vi "PMT imaging_ v2.vi"() -> ()   [LabVIEW 2012]
uses:
  <vilib>/DAQmx/write.llb/DAQmx Write (Analog 1D Wfm NChan NSamp).vi
  <vilib>/DAQmx/read.llb/DAQmx Read (Counter 1D U32 1Chan NSamp).vi
  <vilib>/DAQmx/create/channels.llb/DAQmx Create Channel (AO-Voltage-Basic).vi
  <vilib>/DAQmx/configure/timing.llb/DAQmx Timing (Sample Clock).vi
  <vilib>/DAQmx/configure/trigger.llb/DAQmx Start Trigger (Digital Edge).vi
  <vilib>/DAQmx/create/channels.llb/DAQmx Create Channel (CI-Count Edges).vi
  <vilib>/DAQmx/miscellaneous.llb/DAQmx Fill In Error Info.vi
  <resource>/objmgr/daqmx.rc
panel:
  in  "shift":i8
  in  "String":string
  out "Image original":T1(plugin-control)
  in  "Slices":i32
  in  "Step size(um)":dbl
  in  "Normalization":dbl=255.0
  out "Output":dbl[](array[numeric])
  out "size(s)":i32
  out "data":u32[](array[numeric])
  out "image normalize":T1(plugin-control)
  in  "Exp Time (s)":dbl=4.0
  in  "Y line":i32=512
  in  "Y step (um)":dbl=0.1
  in  "X step (um)":dbl=0.1
  in  "X pixel":i32=512
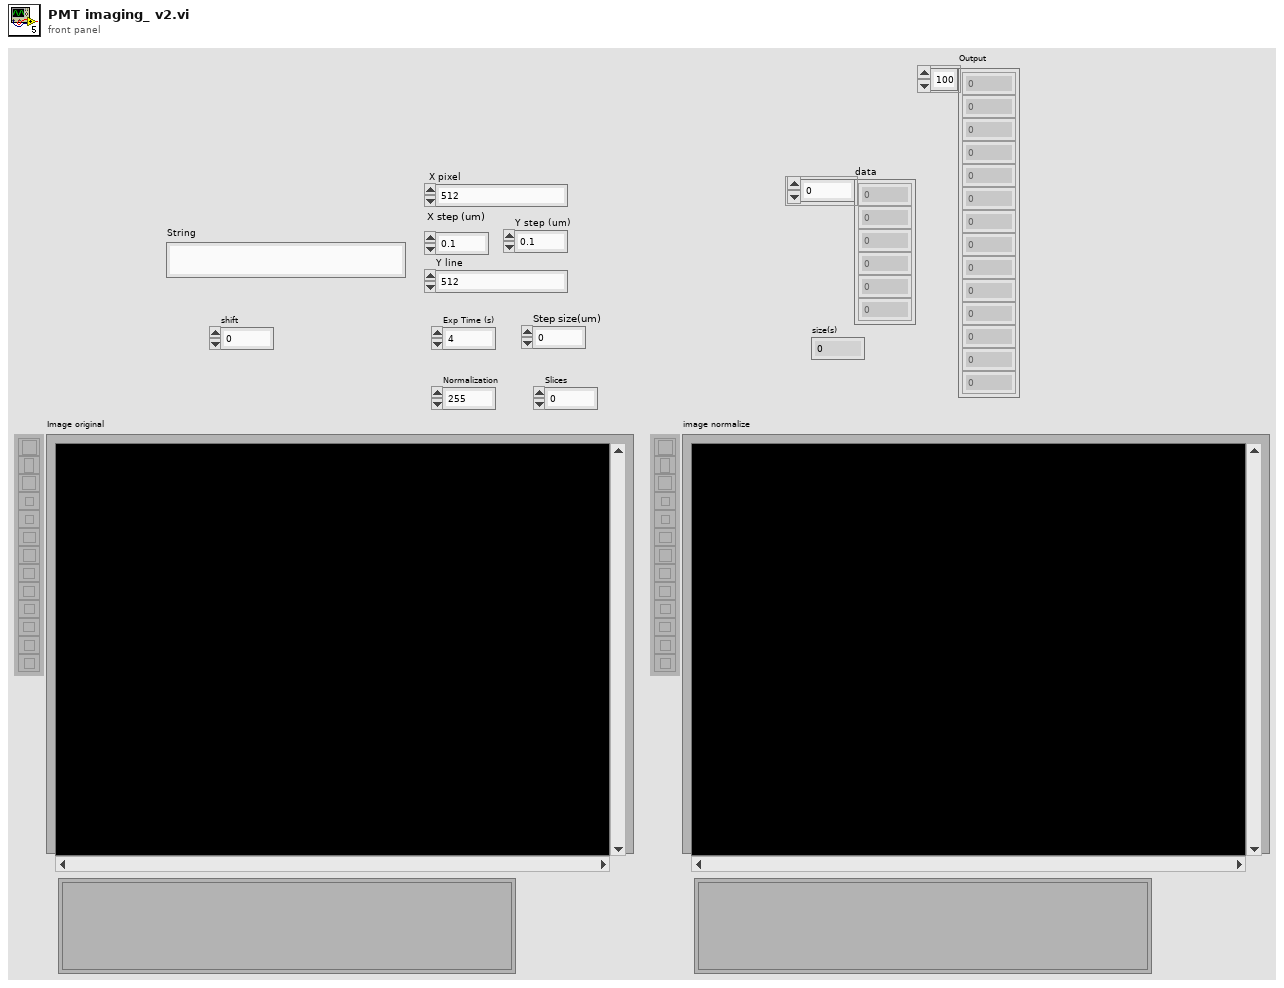
[diagram p1: front panel]
types:
  T1 = typedef "IMAQ Image.ctl" = refnum<image>
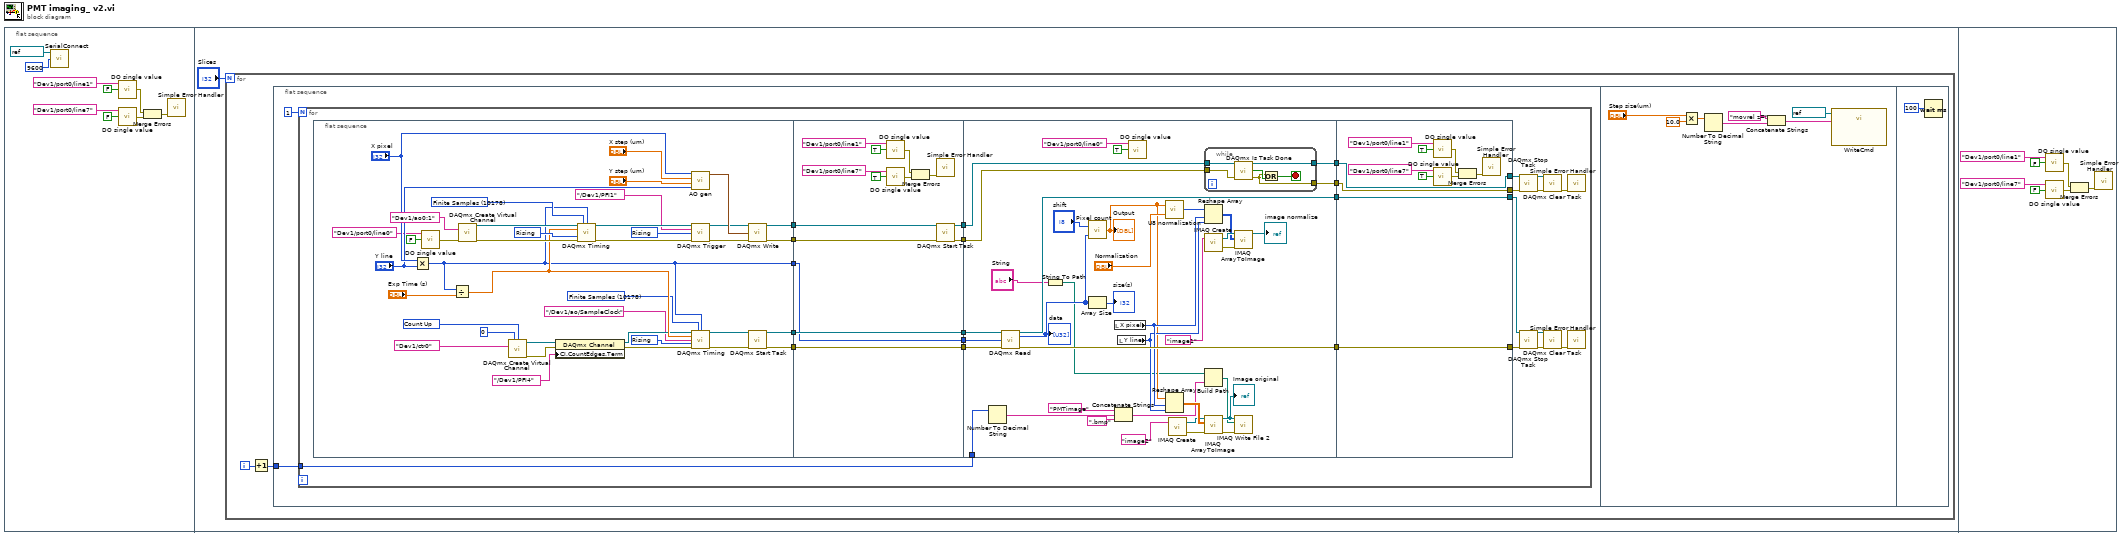
[diagram p0: block diagram]
diagram:
  n1 = flat-sequence {
    frame #0 {
      n2 = call "SerialConnect.vi"("baud rate (9600)"=u32 9600, "VISA resource name"=refnum<visa-resource-name> "COM1") -> ()  [unwired: 1 in, 3 out]
      n3 = call "DO single value.vi"("data"=FALSE, "lines"=tag "Dev1/port0/line1") -> ("error out"=w2:errorcluster)  [unwired: 1 in]
      n4 = call "DO single value.vi"("data"=FALSE, "lines"=tag "Dev1/port0/line7") -> ("error out"=w1:errorcluster)  [unwired: 1 in]
      n5 = Merge Errors(w2, w1) -> (w3:errorcluster)
      n6 = call <vilib>:"Simple Error Handler.vi"("error in (no error)"=w3) -> ()  [unwired: 4 in, 5 out]
    }
    frame #1 {
      n7 = for {
        N: "Slices" -> [_]
        i -> [w12]
        n8 = Increment(x=w12) -> (x+1=w11:i32)
        n9 = flat-sequence {
          tunnel: w11 -> [w13]
          frame #0 {
            n10 = for {
              N: 1 -> [_]
              tunnel: w13 -> [w15]
              n11 = flat-sequence {
                tunnel: [w61] -> w31
                tunnel: [w60] -> w30
                tunnel: [w51] -> w29
                tunnel: [w50] -> w28
                tunnel: [w49] -> w27
                tunnel: [w92] -> w24
                tunnel: [w91] -> w23
                tunnel: [w90] -> w22
                tunnel: [w89] -> w21
                tunnel: [w88] -> w20
                tunnel: w27 -> [w88]
                tunnel: w28 -> [w86]
                tunnel: w29 -> [w87]
                tunnel: w30 -> [w91]
                tunnel: w31 -> [w92]
                tunnel: w24 -> [w124]
                tunnel: w23 -> [w123]
                tunnel: w22 -> [w126]
                tunnel: w21 -> [w125]
                tunnel: w20 -> [w120]
                tunnel: [w122] -> w19
                tunnel: [w121] -> w18
                tunnel: [w128] -> w17
                tunnel: [w127] -> w16
                tunnel: w15 -> [w103]
                tunnel: [w144] -> w36
                tunnel: [w145] -> w37
                tunnel: [w146] -> w38
                tunnel: [w147] -> w39
                tunnel: w19 -> [w147]
                tunnel: w18 -> [w146]
                tunnel: w17 -> [w145]
                tunnel: w16 -> [w144]
                frame #0 {
                  w41 = 10128 items=["Count Up"=10128, "Count Down"=10124, "Externally Controlled"=10326] ("count direction")
                  w42 = 10280 items=["Rising"=10280, "Falling"=10171] ("edge")
                  w65 = 10178 items=["Finite Samples"=10178, "Continuous Samples"=10123, "Hardware Timed Single Point"=12522] ("sample mode")
                  w67 = 10280 items=["Rising"=10280, "Falling"=10171] ("active edge")
                  w69 = 10178 items=["Finite Samples"=10178, "Continuous Samples"=10123, "Hardware Timed Single Point"=12522] ("sample mode")
                  w73 = 10280 items=["Rising"=10280, "Falling"=10171] ("active edge")
                  n12 = Multiply(x="X pixel", y="Y line") -> (x*y=w49:i32)
                  n13 = call "DO single value.vi"("data"=FALSE, "lines"=tag "Dev1/port0/line0") -> ("error out"=w64:errorcluster)  [unwired: 1 in]
                  n14 = Divide(x=w49, y="Exp Time (s)") -> (x/y=w66:dbl)
                  n15 = call-poly <vilib>:"DAQmx Create Virtual Channel.vi"("physical channels"=tag "Dev1/ao0:1", "error in"=w64) -> ("task out"=w74:refnum<k21>, "error out"=w75:errorcluster)  [unwired: 7 in, 5 out]
                  n16 = call-poly <vilib>:"DAQmx Create Virtual Channel.vi"("initial count"=u32 0, "count direction"=w41, "counter"=tag "Dev1/ctr0") -> ("task out"=w58:refnum<k21>, "error out"=w57:errorcluster)  [unwired: 4 in, 7 out]
                  n17 = property class="DAQmx Channel"(reference=w58, error in=w57, "CI.CountEdges.Term"=tag "/Dev1/PFI4") -> (reference out=w55:refnum<k21>, error out=w54:errorcluster)
                  n18 = call-poly <vilib>:"DAQmx Timing.vi"("task/channels in"=w74, "sample mode"=w69, "samples per channel"=w49, "rate"=w66, "active edge"=w73, "error in"=w75) -> ("task out"=w47:refnum<k21>, "error out"=w46:errorcluster)  [unwired: 1 in, 7 out]
                  n19 = call "AO gen.vi"("X pixel"="X pixel", "X step (um)"="X step (um)", "Y step (um)"="Y step (um)", "Y line"="Y line") -> ("waveform output"=w68:waveform(dbl)[])  [unwired: 2 in, 1 out]
                  n20 = call-poly <vilib>:"DAQmx Trigger.vi"("task/channels in"=w47, "source"=tag "/Dev1/PFI1", "edge"=w42, "error in"=w46) -> ("task out"=w45:refnum<k21>, "error out"=w44:errorcluster)  [unwired: 10 in]
                  n21 = call-poly <vilib>:"DAQmx Timing.vi"("task/channels in"=w55, "sample mode"=w65, "samples per channel"=w49, "rate"=w66, "source"=tag "/Dev1/ao/SampleClock", "active edge"=w67, "error in"=w54) -> ("task out"=w53:refnum<k21>, "error out"=w52:errorcluster)  [unwired: 7 out]
                  n22 = call-poly <vilib>:"DAQmx Write.vi"("task/channels in"=w45, "data"=w68, "error in"=w44) -> ("task out"=w51:refnum<k21>, "error out"=w50:errorcluster)  [unwired: 2 in, 9 out]
                  n23 = call <vilib>:"DAQmx Start Task.vi"("task/channels in"=w53, "error in"=w52) -> ("task out"=w61:refnum<k21>, "error out"=w60:errorcluster)  [unwired: 12 out]
                }
                frame #1 {
                  n24 = call "DO single value.vi"("data"=TRUE, "lines"=tag "Dev1/port0/line1") -> ("error out"=w80:errorcluster)  [unwired: 1 in]
                  n25 = call "DO single value.vi"("data"=TRUE, "lines"=tag "Dev1/port0/line7") -> ("error out"=w79:errorcluster)  [unwired: 1 in]
                  n26 = Merge Errors(w80, w79) -> (w81:errorcluster)
                  n27 = call <vilib>:"Simple Error Handler.vi"("error in (no error)"=w81) -> ()  [unwired: 4 in, 5 out]
                  n28 = call <vilib>:"DAQmx Start Task.vi"("task/channels in"=w87, "error in"=w86) -> ("task out"=w90:refnum<k21>, "error out"=w89:errorcluster)  [unwired: 12 out]
                }
                frame #2 {
                  n29 = Number To Decimal String(number=w103) -> (decimal integer string=w102:string)  [unwired: 1 in]
                  n30 = call-poly <vilib>:"DAQmx Read.vi"("task/channels in"=w124, "number of samples per channel"=w120, "error in"=w123) -> ("task out"=w122:refnum<k21>, "data"=w115:u32[], "error out"=w121:errorcluster)  [unwired: 10 in]
                  "data" <- w115
                  n31 = String To Path(string="String") -> (path=w94:path)
                  n32 = call "Pixel count.vi"("Input"=w115, "shift"="shift") -> ("Output"=w108:dbl[])
                  "Output" <- w108
                  n33 = Array Size(array=w115) -> (size(s)=→"size(s)":i32)
                  n34 = local read "X pixel"() -> (w110:i32)
                  n35 = Concatenate Strings("PMTimage" ("string"), w102, ".bmp" ("string")) -> (w99:string)
                  n36 = local read "Y line"() -> (w109:i32)
                  n37 = call "DO single value.vi"("data"=TRUE, "lines"=tag "Dev1/port0/line0") -> ()  [unwired: 1 in, 1 out]
                  n38 = call "U8 normalization.vi"("Max"="Normalization", "Input"=w108) -> ("Output"=w112:u8[])
                  n39 = Reshape Array(w108, w110, w109) -> (w107:dbl[][])
                  n40 = call "IMAQ Create"("Image Name"="image2") -> ("New Image"=w106:T1, "error out"=w105:errorcluster)  [unwired: 4 in]
                  n41 = while {
                    tunnel: [w134] -> w128
                    tunnel: [w133] -> w127
                    tunnel: w126 -> [w132]
                    tunnel: w125 -> [w131]
                    stop <- w135 stop-if-true
                    n42 = call <vilib>:"DAQmx Is Task Done.vi"("task/channels in"=w132, "error in"=w131) -> ("task out"=w134:refnum<k21>, "task done?"=w136:bool, "error out"=w133:errorcluster)  [unwired: 11 in]
                    n43 = Or(x=w133, y=w136) -> (x .or. y?=w135:bool)
                  }
                  n44 = Reshape Array(w112, w110, w109) -> (w113:u8[][])
                  n45 = call "IMAQ Create"("Image Name"="image1") -> ("New Image"=w119:T1, "error out"=w118:errorcluster)  [unwired: 4 in]
                  n46 = Build Path(base path=w94, name or relative path=w99) -> (appended path=w98:path)
                  n47 = call "IMAQ ArrayToImage"("error in (no error)"=w105, "Image Pixels (U8)"=w107, "Image"=w106) -> ("error out"=w97:errorcluster, "Image Out"=w104:T1)  [unwired: 7 in]
                  "Image original" <- w104
                  n48 = call "IMAQ ArrayToImage"("error in (no error)"=w118, "Image Pixels (U8)"=w113, "Image"=w119) -> ("Image Out"=→"image normalize":T1)  [unwired: 7 in, 1 out]
                  n49 = call-poly "IMAQ Write File 2"("error in (no error)"=w97, "File Path"=w98, "Image"=w104) -> ()  [unwired: 7 in, 2 out]
                }
                frame #3 {
                  n50 = call "DO single value.vi"("data"=TRUE, "lines"=tag "Dev1/port0/line1") -> ("error out"=w138:errorcluster)  [unwired: 1 in]
                  n51 = call "DO single value.vi"("data"=TRUE, "lines"=tag "Dev1/port0/line7") -> ("error out"=w137:errorcluster)  [unwired: 1 in]
                  n52 = Merge Errors(w138, w137) -> (w139:errorcluster)
                  n53 = call <vilib>:"Simple Error Handler.vi"("error in (no error)"=w139) -> ()  [unwired: 4 in, 5 out]
                }
              }
              n54 = call <vilib>:"DAQmx Stop Task.vi"("task/channels in"=w37, "error in"=w36) -> ("task out"=w33:refnum<k21>, "error out"=w32:errorcluster)  [unwired: 12 out]
              n55 = call <vilib>:"DAQmx Stop Task.vi"("task/channels in"=w39, "error in"=w38) -> ("task out"=w34:refnum<k21>, "error out"=w35:errorcluster)  [unwired: 12 out]
              n56 = call <vilib>:"DAQmx Clear Task.vi"("task in"=w33, "error in"=w32) -> ("error out"=w26:errorcluster)  [unwired: 13 in]
              n57 = call <vilib>:"DAQmx Clear Task.vi"("task in"=w34, "error in"=w35) -> ("error out"=w25:errorcluster)  [unwired: 13 in]
              n58 = call <vilib>:"Simple Error Handler.vi"("error in (no error)"=w26) -> ()  [unwired: 4 in, 5 out]
              n59 = call <vilib>:"Simple Error Handler.vi"("error in (no error)"=w25) -> ()  [unwired: 4 in, 5 out]
            }
          }
          frame #1 {
            n60 = Multiply(x="Step size(um)", y=10.0) -> (x*y=w153:dbl)
            n61 = Number To Decimal String(number=w153) -> (decimal integer string=w150:string)  [unwired: 1 in]
            n62 = Concatenate Strings("movrel z=", w150) -> (w151:string)
            n63 = call "WriteCmd.vi"("Command"=w151, "VISA resource name"=refnum<visa-resource-name> "COM1") -> ()  [unwired: 1 in, 1 out]
          }
          frame #2 {
            n64 = Wait (ms)(milliseconds to wait=u32 100) -> ()  [unwired: 1 out]
          }
        }
      }
    }
    frame #2 {
      n65 = call "DO single value.vi"("data"=FALSE, "lines"=tag "Dev1/port0/line1") -> ("error out"=w157:errorcluster)  [unwired: 1 in]
      n66 = call "DO single value.vi"("data"=FALSE, "lines"=tag "Dev1/port0/line7") -> ("error out"=w156:errorcluster)  [unwired: 1 in]
      n67 = Merge Errors(w157, w156) -> (w158:errorcluster)
      n68 = call <vilib>:"Simple Error Handler.vi"("error in (no error)"=w158) -> ()  [unwired: 4 in, 5 out]
    }
  }
